vi "Indentation GUI - v4.vi"() -> ()   [LabVIEW 2013]
uses:
  Program Files (x86)/National Instruments/LabVIEW 2013/examples/Instrument IO/Serial/Serial - XON-XOFF Characters.ctl
  Program Files (x86)/National Instruments/LabVIEW 2013/examples/Instrument IO/Serial/Serial - ASCII Characters.ctl
  Program Files (x86)/National Instruments/LabVIEW 2013/examples/Instrument IO/Serial/Serial - Settings.ctl
  <vilib>/Instr/_visa.llb/VISA Configure Serial Port (Instr).vi
  <userlib>/DAQNavi Polymorphic VI/create/DAQNavi Create Channel(AI-Voltage).vi
  <userlib>/DAQNavi Polymorphic VI/read/DAQNavi Read (Analog DBL 1Chan 1Samp).vi
  <vilib>/Utility/file.llb/Write To Spreadsheet File (DBL).vi
panel:
  in  "offset":dbl
  in  "ground distance":dbl
  in  "contact":bool
  in  "停止 6":bool
  out "运动命令执行串口响应 4":string
  in  "终止符时结束读取？ 8":bool=TRUE
  in  "XON/XOFF字符 8":T1={"XON"=enum."DC1", "XOFF"=enum."DC3"}
  in  "终止符时结束写入？ 8":bool=TRUE
  in  "终止符 8":u8=10 format="%.0x"
  out "坐标设定命令串口传输响应 4":string
  in  "终止符时结束读取？ 7":bool=TRUE
  in  "XON/XOFF字符 7":T1={"XON"=enum."DC1", "XOFF"=enum."DC3"}
  in  "终止符时结束写入？ 7":bool=TRUE
  in  "终止符 7":u8=10 format="%.0x"
  in  "Fast Move":bool
  in  "停止 5":bool
  out "运动命令执行串口响应 3":string
  in  "终止符时结束读取？ 6":bool=TRUE
  in  "XON/XOFF字符 6":T1={"XON"=enum."DC1", "XOFF"=enum."DC3"}
  in  "终止符时结束写入？ 6":bool=TRUE
  in  "终止符 6":u8=10 format="%.0x"
  out "坐标设定命令串口传输响应 3":string
  in  "终止符时结束读取？ 5":bool=TRUE
  in  "XON/XOFF字符 5":T1={"XON"=enum."DC1", "XOFF"=enum."DC3"}
  in  "终止符时结束写入？ 5":bool=TRUE
  in  "终止符 5":u8=10 format="%.0x"
  in  "Backoff":bool
  in  "Sample+Slide":dbl
  in  "BaseLine":dbl=1.86
  in  "停止 4":bool
  out "运动命令执行串口响应 2":string
  in  "终止符时结束读取？ 4":bool=TRUE
  in  "XON/XOFF字符 4":T1={"XON"=enum."DC1", "XOFF"=enum."DC3"}
  in  "终止符时结束写入？ 4":bool=TRUE
  in  "终止符 4":u8=10 format="%.0x"
  out "Position setup command \nseries transport response 2":string
  in  "终止符时结束读取？ 3":bool=TRUE
  in  "XON/XOFF字符 3":T1={"XON"=enum."DC1", "XOFF"=enum."DC3"}
  in  "终止符时结束写入？ 3":bool=TRUE
  in  "终止符 3":u8=10 format="%.0x"
  out "Delay Counter":u64
  in  "indentation":bool
  in  "终止符 2":u8=10 format="%.0x"
  in  "终止符时结束写入？ 2":bool=TRUE
  in  "XON/XOFF字符 2":T1={"XON"=enum."DC1", "XOFF"=enum."DC3"}
  in  "终止符时结束读取？ 2":bool=TRUE
  out "Position setup command \nseries transport response":string
  in  "停止 3":bool
  out "Movement command execute \nseries transport response":string
  in  "停止 2":bool
  out "电压":cluster{"data":dbl, "data":dbl}(graph)
  out "data acquistion":bool
  in  "file path (dialog if empty)":path=path "C:/Users/user/Desktop/indentation data/新建 Microsoft Office Excel 工作表.xls" caption="文件路径 File Path"
  in  "Dwell Time (s)":dbl=180.0
  in  "Sample Frequency (Hz)":dbl=1000.0
  in  "Displacement (mm)":dbl
  in  "终止符时结束读取？":bool=TRUE
  in  "XON/XOFF字符":T1={"XON"=enum."DC1", "XOFF"=enum."DC3"}
  in  "终止符时结束写入？":bool=TRUE
  in  "终止符":u8=10 format="%.0x"
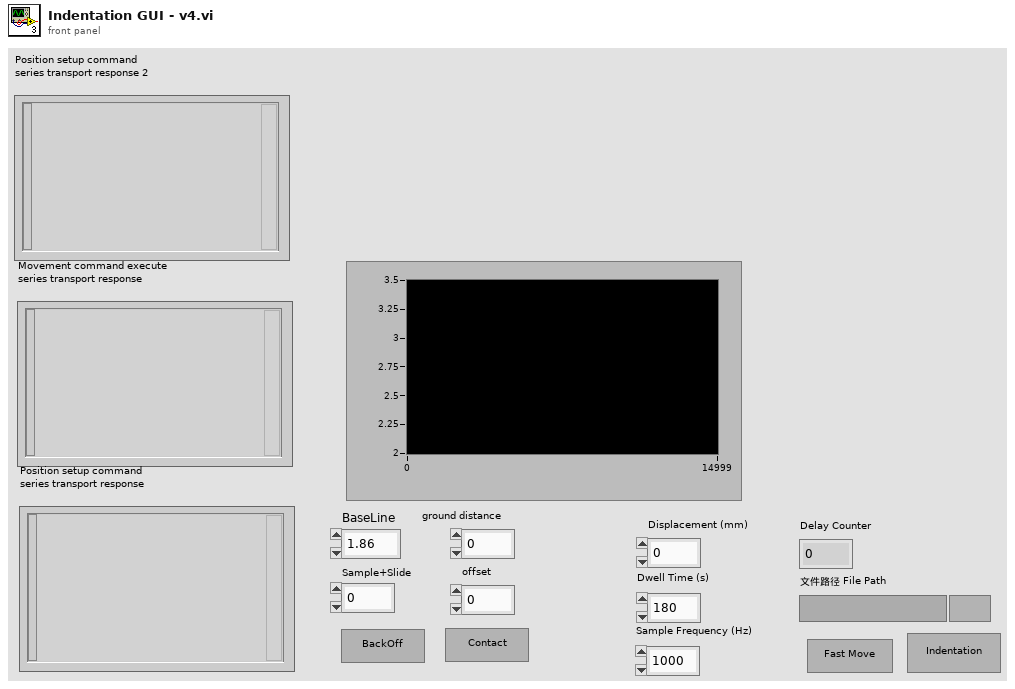
[diagram p1: front panel]
types:
  T1 = typedef "Serial - XON-XOFF Characters.ctl" = cluster{"XON":T2, "XOFF":T2}
  T2 = typedef "Serial - ASCII Characters.ctl" = enum16{"NUL", "SOH", "STX", "ETX", "EOT", "ENQ", "ACK", "BEL", "BS", "HT", "LF", "VT", "FF", "CR", "SO", "SI", "DLE", "DC1", "DC2", "DC3", "DC4", "NAK", "SYN", "ETB", "CAN", "EM", "SUB", "ESC", "FS", "GS", "RS", "US", "SP", "!", "\"", "#", "$", "%", "&", "'", "(", ")", "*", "+", ",", "- (-)", ".", "/", "0", "1", "2", "3", "4", "5", "6", "7", "8", "9", ":", ";", "<", "=", ">", "?", "@", "A", "B", "C", "D", "E", "F", "G", "H", "I", "J", "K", "L", "M", "N", "O", "P", "Q", "R", "S", "T", "U", "V", "W", "X", "Y", "Z", "[", "\\", "]", "^", "_", "`", "a", "b", "c", "d", "e", "f", "g", "h", "i", "j", "k", "l", "m", "n", "o", "p", "q", "r", "s", "t", "u", "v", "w", "x", "y", "z", "{", "|", "}", "~"}
  T3 = typedef "Serial - Settings.ctl" = cluster{"波特率":u32, "数据比特":u16, "奇偶":enum16{"None", "Odd", "Even", "Mark", "Space"}, "停止位":u16, "流控制":u16}
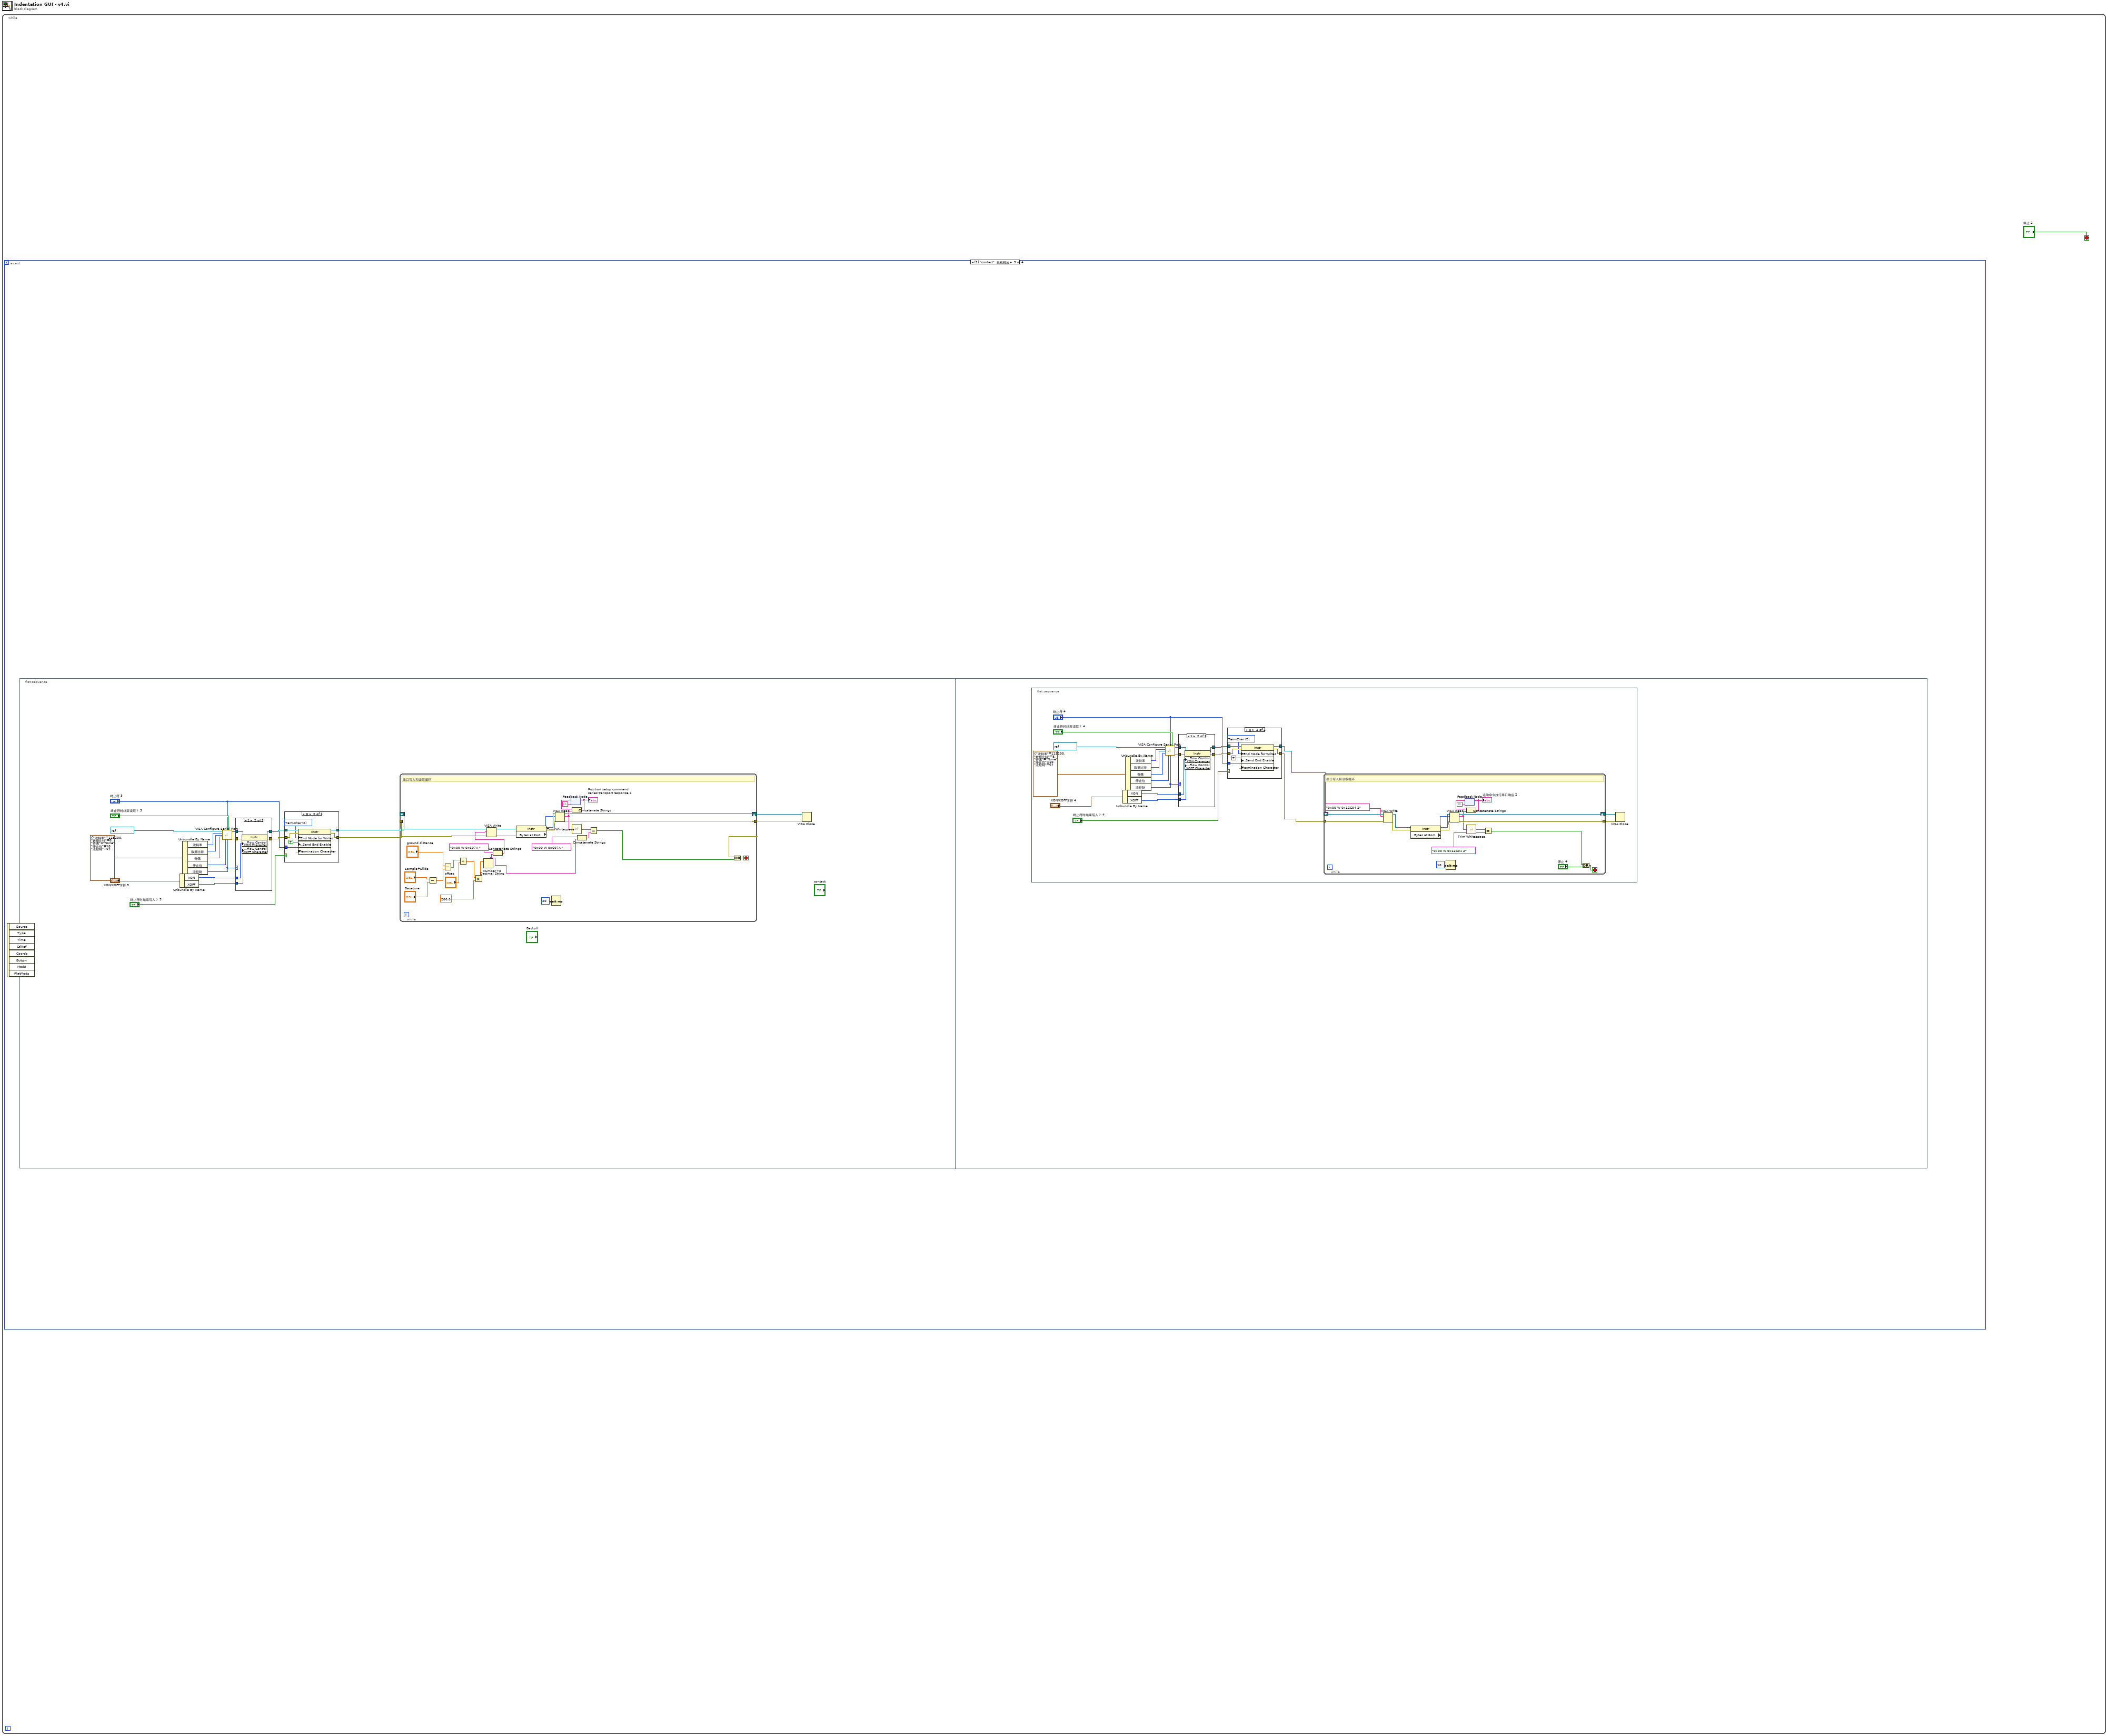
[diagram p0: block diagram]
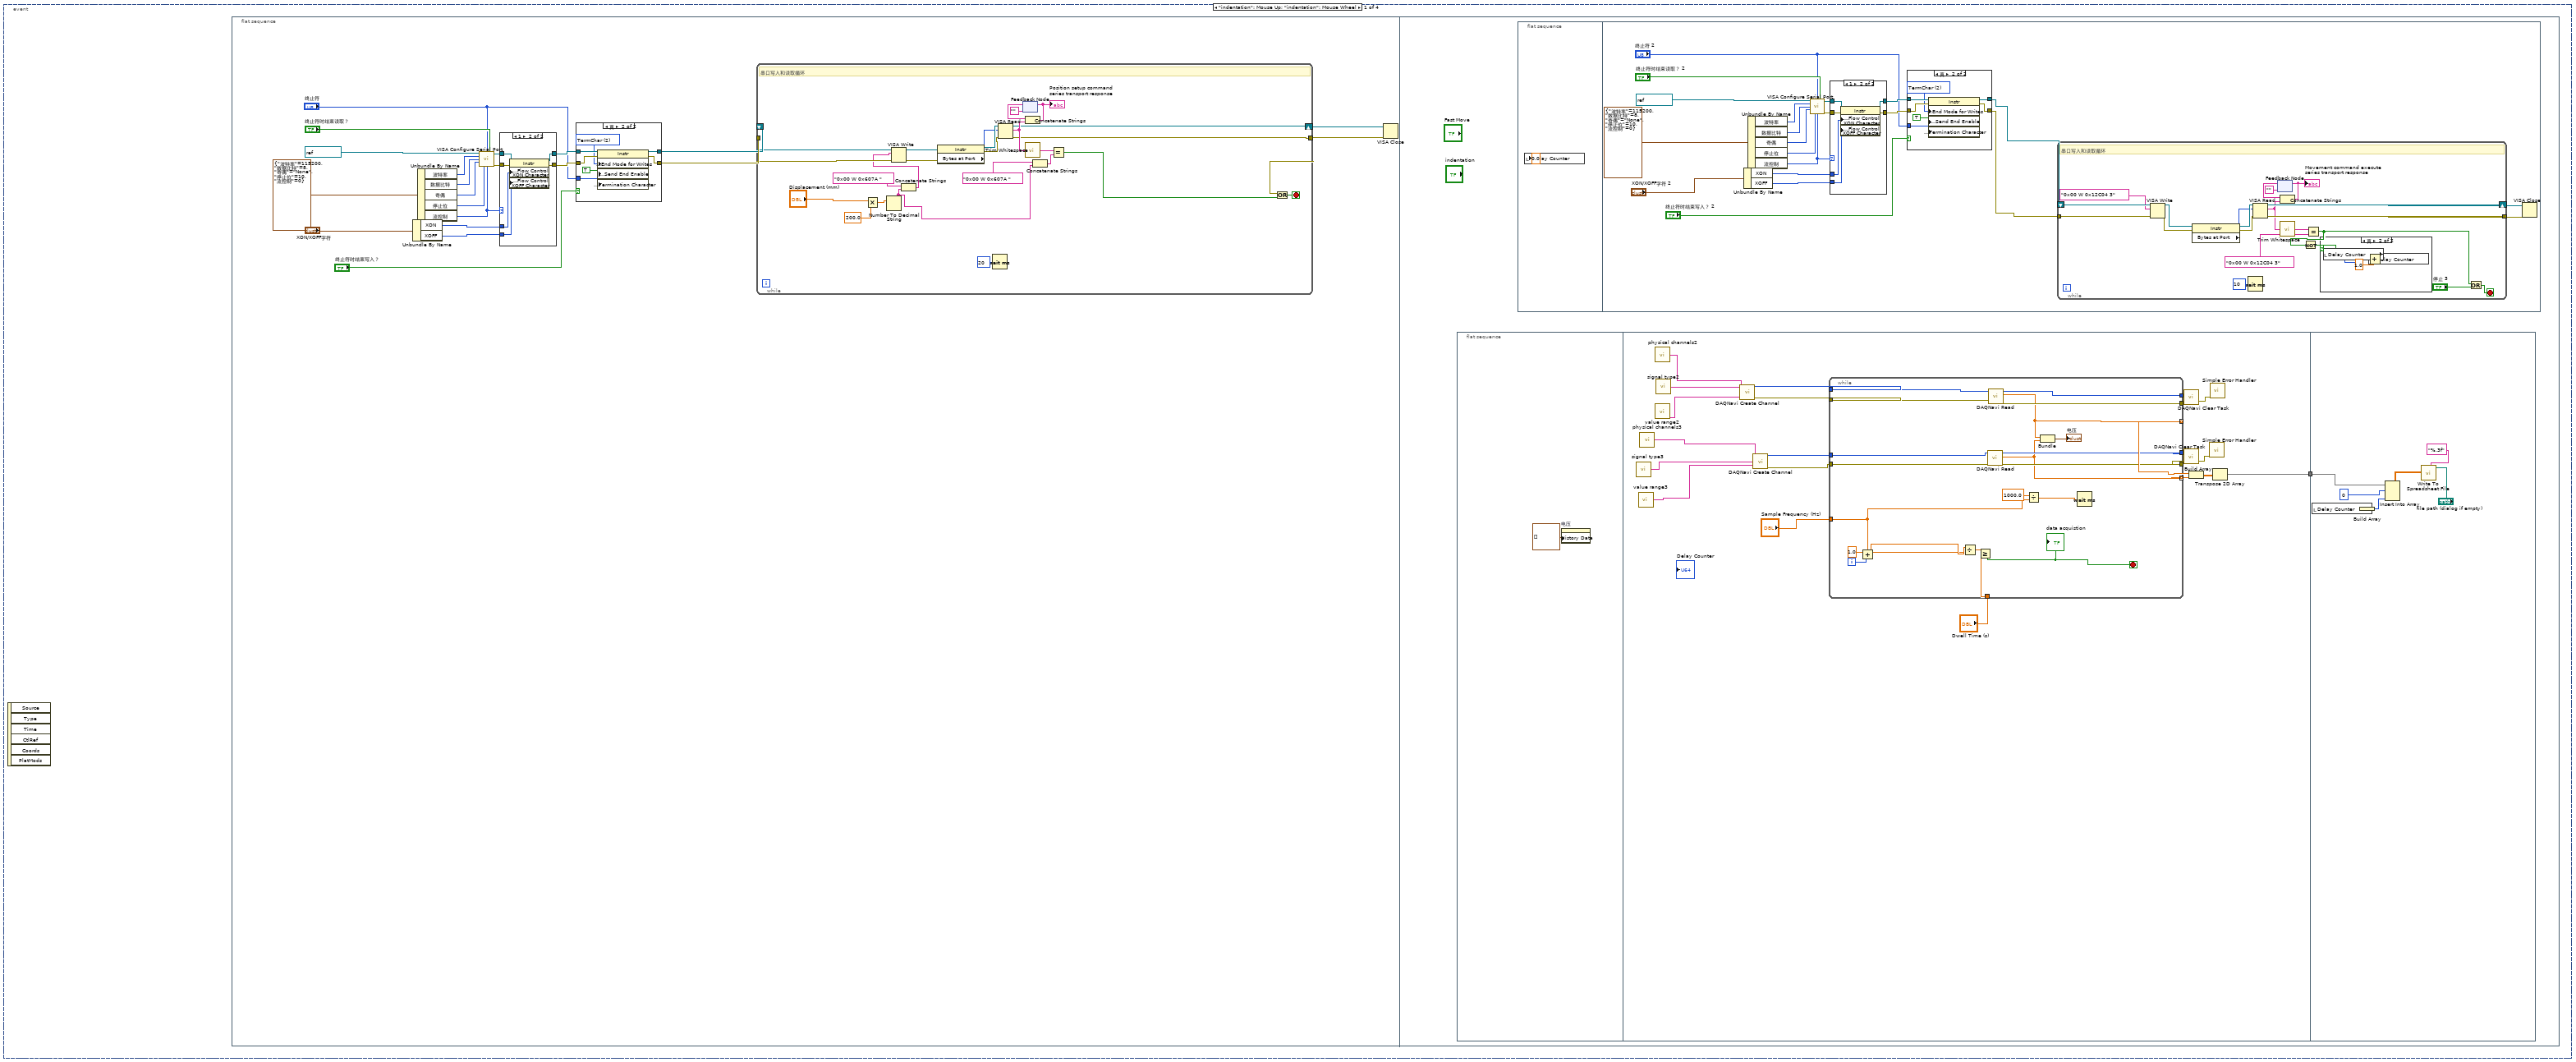
[diagram p2: hidden frame]
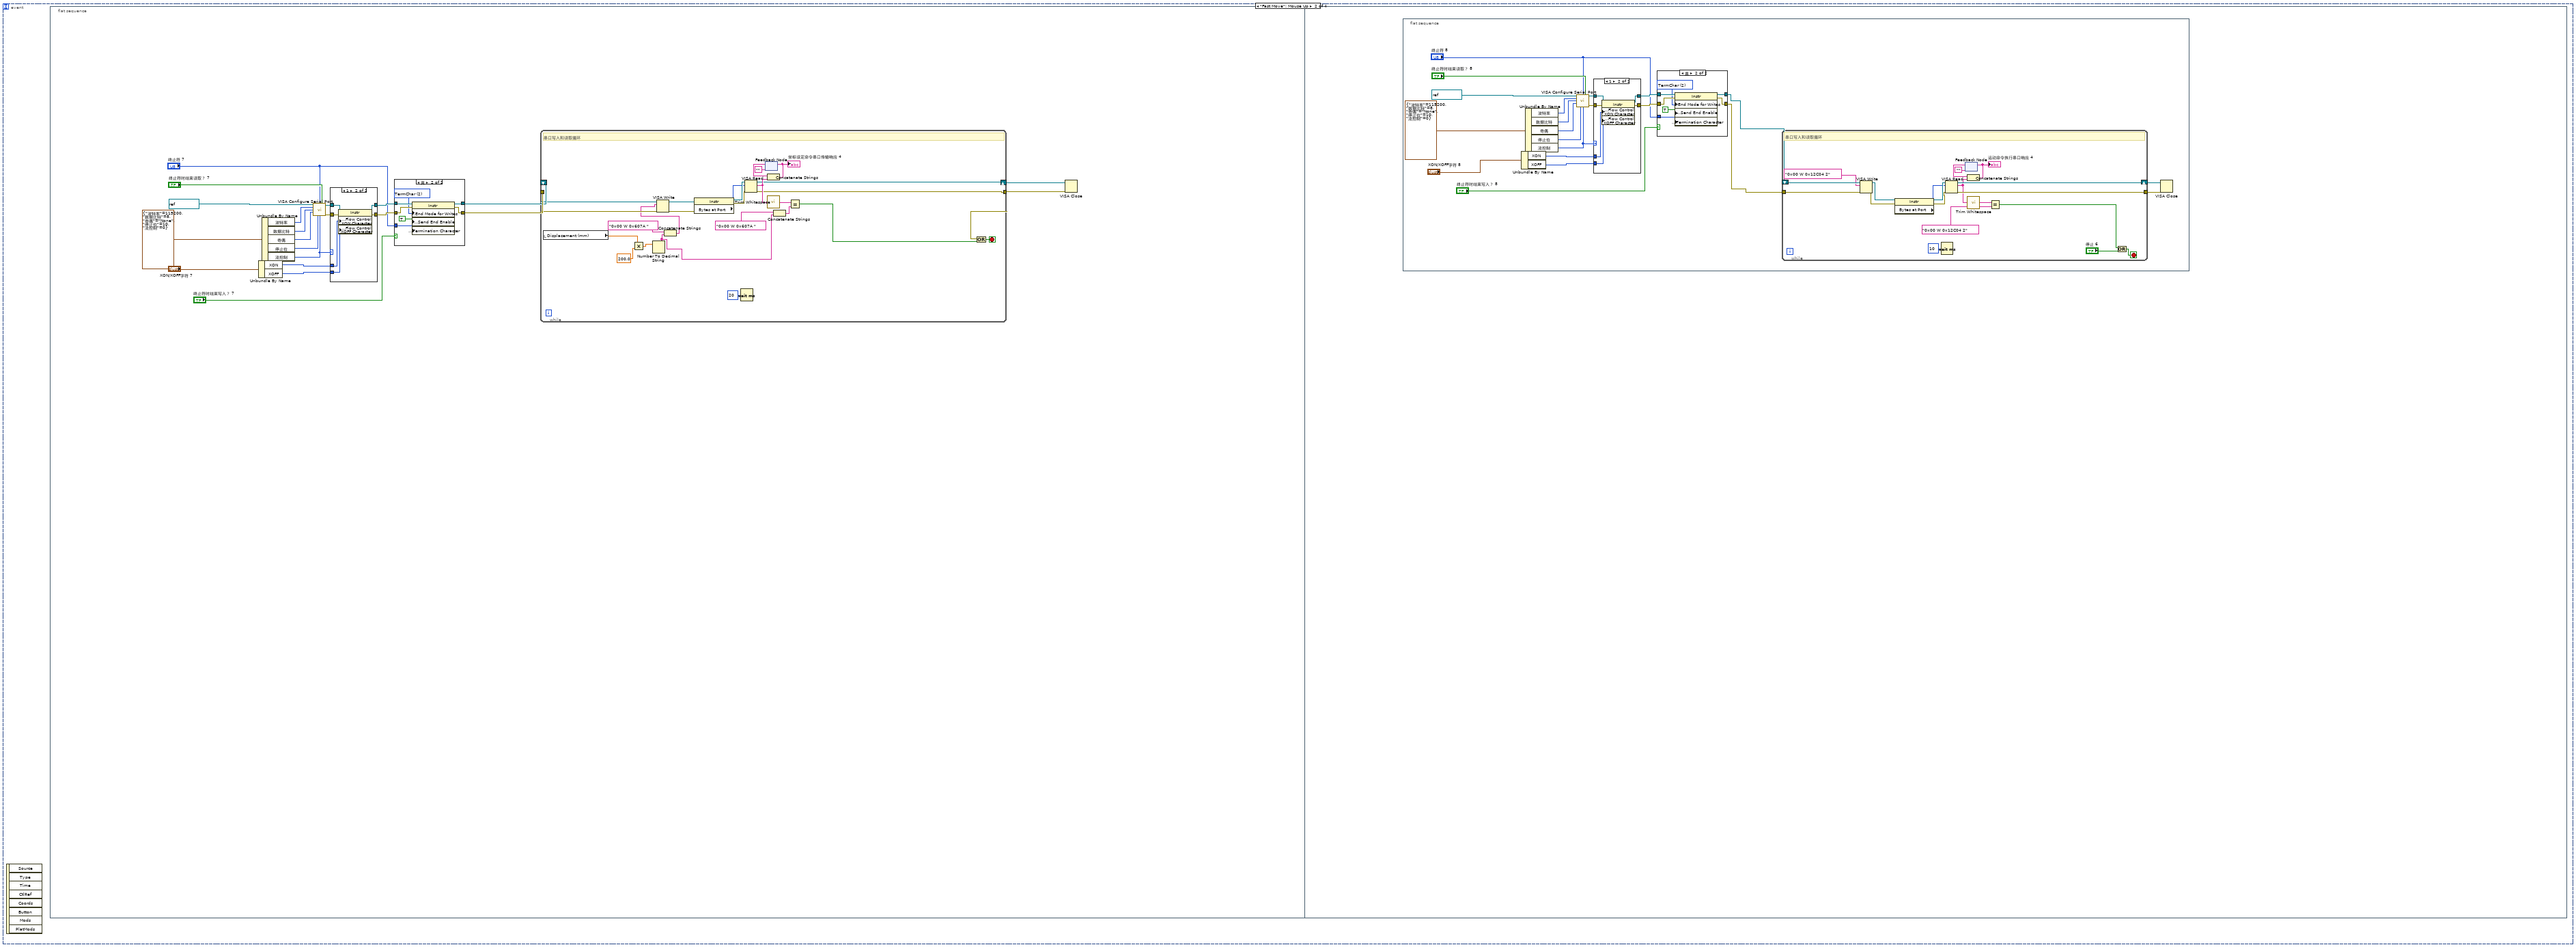
[diagram p8: hidden frame]
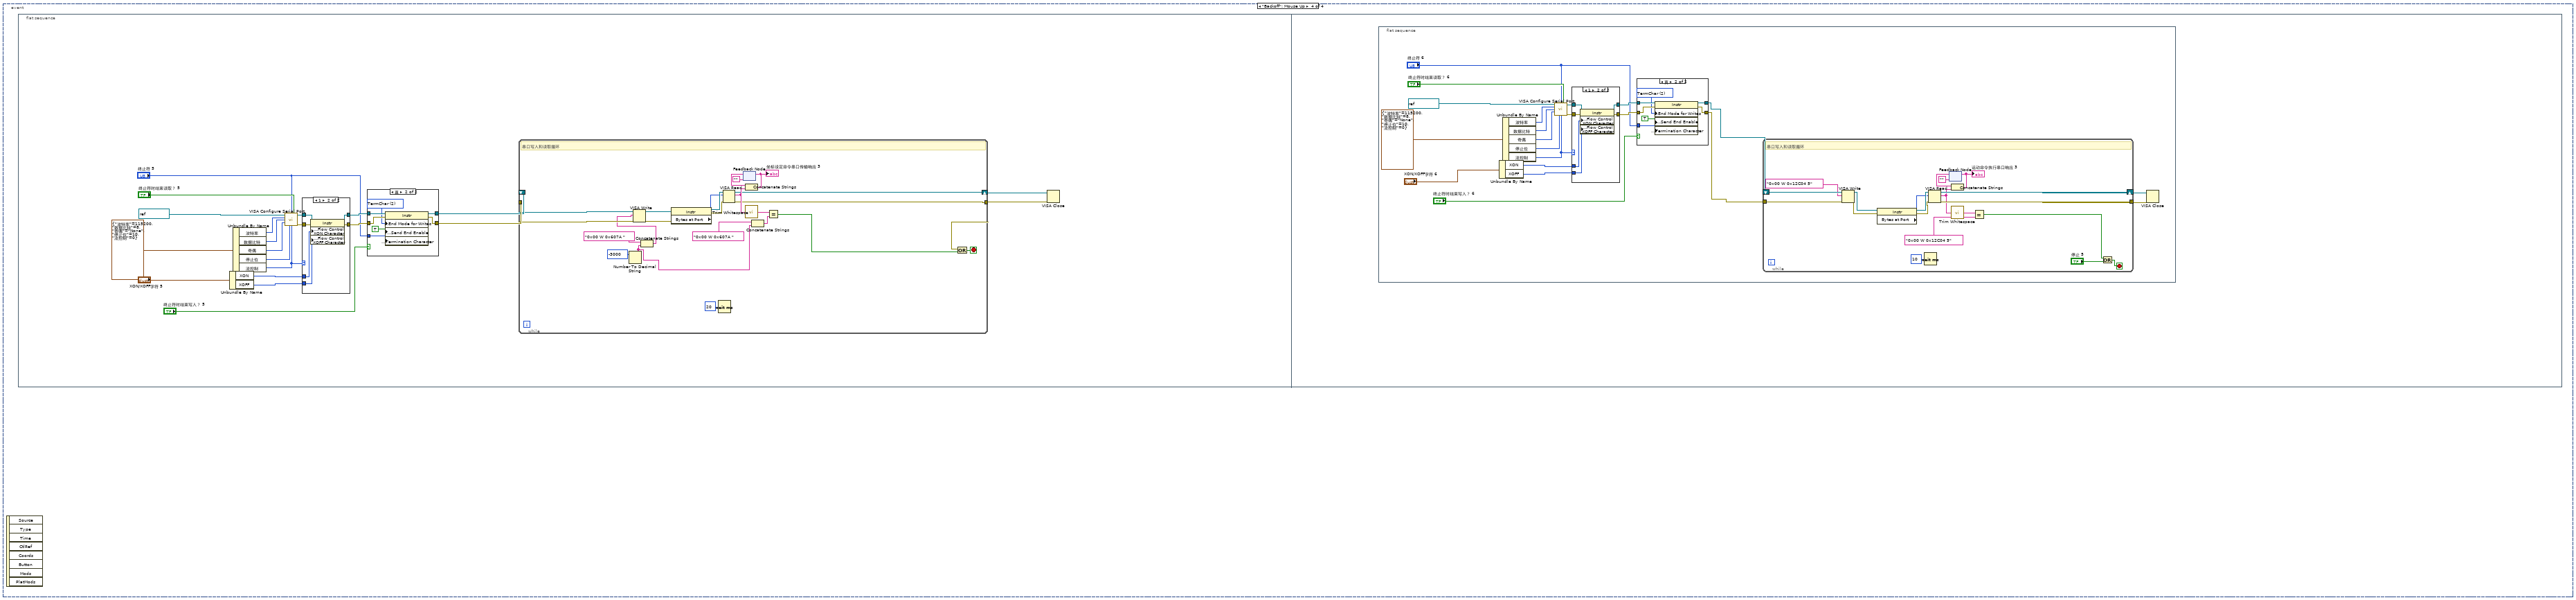
[diagram p17: hidden frame]
diagram:
  n1 = while {
    stop <- "停止 2" stop-if-true
    n2 = event shown="[2] \"contact\": 鼠标释放" {
      selector: _ -> [_ _ _ _]
      dyn-events: _ -> [_ _ _ _]
      timeout: _ -> [_ _ _ _]
      event "indentation": Mouse Up; "indentation": Mouse Wheel {
        n3 = event-data() -> ()  [unwired: 1 in, 6 out]
        n4 = flat-sequence {
          frame #0 {
            n5 = Unbundle By Name("XON/XOFF字符") -> ("XON"=w11:T2, "XOFF"=w10:T2)
            n6 = Unbundle By Name(T3 {"波特率"=115200, "数据比特"=8, "奇偶"=enum."None", "停止位"=10, "流控制"=0} ("串口设置")) -> ("波特率"=w15:u32, "数据比特"=w16:u16, "奇偶"=w17:enum16{"None", "Odd", "Even", "Mark", "Space"}, "停止位"=w18:u16, "流控制"=w12:u16)
            n7 = call-poly "VISA Configure Serial Port"("VISA resource name"=refnum<visa-resource-name> "COM3" ("VISA资源名称"), "termination char\n(0xA = '\\n' = LF)"="终止符", "Enable Termination\nChar (T)"="终止符时结束读取？", "baud rate (9600)"=w15, "data bits (8)"=w16, "parity (0:none)"=w17, "stop bits (10: 1 bit)"=w18, "flow control (0:none)"=w12) -> ("VISA resource name out"=w19:refnum<visa-resource-name>, "error out"=w20:errorcluster)  [unwired: 2 in, 4 out]
            n8 = case shown="1" w12 {
              tunnel: [w32 w39] -> w9
              tunnel: [w33 w38] -> w7
              tunnel: w20 -> [w32 w37]
              tunnel: w19 -> [w33 w36]
              tunnel: w11 -> [_ w35]
              tunnel: w10 -> [_ w34]
              frame Default {
              }
              frame 1 {
                n9 = property class="Instr"(reference=w36, error in=w37, "Serial Settings:Flow Control XON Character"=w35, "Serial Settings:Flow Control XOFF Character"=w34) -> (reference out=w38:refnum<visa-resource-name>, error out=w39:errorcluster)
              }
            }
            n10 = case shown="真" "终止符时结束写入？" {
              tunnel: w7 -> [w23 w31]
              tunnel: w9 -> [w24 w30]
              tunnel: [w23 w29] -> w6
              tunnel: [w24 w28] -> w8
              tunnel: "终止符" -> [_ w26]
              frame False {
              }
              frame True {
                w27 = u16 2 items=["None", "LastBit", "TermChar", "Break"] ("Serial Settings:Serial End Mode for Writes")
                n11 = property class="Instr"(reference=w31, error in=w30, "Serial Settings:End Mode for Writes"=w27, "Message Based Settings:Send End Enable"=TRUE, "Message Based Settings:Termination Character"=w26) -> (reference out=w29:refnum<visa-resource-name>, error out=w28:errorcluster)
              }
            }
            n12 = while {
              shift-right: [w47] -> w3
              shift-left: w6 -> [w63]
              tunnel: w8 -> [w62]
              tunnel: [w46] -> w2
              stop <- w64 stop-if-true
              # "串口写入和读取循环"
              n13 = Multiply(x="Displacement (mm)", y=200.0) -> (x*y=w59:dbl)
              n14 = Number To Decimal String(number=w59) -> (decimal integer string=w41:string)  [unwired: 1 in]
              n15 = Concatenate Strings("0x00 W 0x607A " ("字符串"), w41) -> (w57:string)
              n16 = VISA Write(VISA resource name=w63, write buffer=w57, error in (no error)=w62) -> (VISA resource name out=w44:refnum<visa-resource-name>, error out=w43:errorcluster)  [unwired: 1 out]
              n17 = property class="Instr"(reference=w44, error in=w43) -> (reference out=w52:refnum<visa-resource-name>, error out=w51:errorcluster, "Bytes at Port"=w50:u32)
              n18 = Wait (ms)(milliseconds to wait=u32 20 ("等待时间（毫秒）")) -> ()  [unwired: 1 out]
              n19 = VISA Read(VISA resource name=w52, byte count=w50, error in (no error)=w51) -> (VISA resource name out=w47:refnum<visa-resource-name>, read buffer=w49:string, error out=w46:errorcluster)  [unwired: 1 out]
              n20 = feedback #1("") -> (w55:string)
              n21 = Concatenate Strings(w55, w49) -> (w54:string)
              "Position setup command \nseries transport response" <- w54
              n22 = feedback-in #1(w54) -> ()
              n23 = call <vilib>:"Trim Whitespace.vi"("string"=w49) -> ("trimmed string"=w48:string)  [unwired: 1 in]
              n24 = Concatenate Strings("0x00 W 0x607A ", w41) -> (w40:string)
              n25 = Equal?(x=w48, y=w40) -> (x = y?=w45:bool)
              n26 = Or(x=w46, y=w45) -> (x .or. y?=w64:bool)
            }
            n27 = VISA Close(VISA resource name=w3, error in (no error)=w2) -> ()  [unwired: 1 out]
          }
          frame #1 {
            n28 = flat-sequence {
              tunnel: [w67] -> w65
              tunnel: w65 -> [w113]
              frame #0 {
                n29 = property on="电压" class="WFChart (严格)"("History Data"=cluster{"data":dbl, "data":dbl}[] [] ("历史数据")) -> ()  [unwired: 2 in, 2 out]
              }
              frame #1 {
                n30 = call "signal type3"() -> ("property value"=w79:string)  [unwired: 1 out]
                n31 = call "value range3"() -> ("property value"=w80:string)  [unwired: 1 out]
                n32 = call "physical channels3"() -> ("property value"=w78:string)  [unwired: 1 out]
                n33 = call "physical channels2"() -> ("property value"=w74:string)  [unwired: 1 out]
                n34 = call "value range2"() -> ("property value"=w75:string)  [unwired: 1 out]
                n35 = call "signal type2"() -> ("property value"=w68:string)  [unwired: 1 out]
                n36 = call-poly <userlib>:"DAQNavi Create Channel.vi"("physical channels"=w74, "signal type"=w68, "value range"=w75) -> ("task out"=w72:i32, "error out"=w71:errorcluster)  [unwired: 2 in, 9 out]
                n37 = call-poly <userlib>:"DAQNavi Create Channel.vi"("physical channels"=w78, "signal type"=w79, "value range"=w80) -> ("task out"=w76:i32, "error out"=w77:errorcluster)  [unwired: 11 in]
                n38 = while {
                  tunnel: w72 -> [w108]
                  tunnel: w71 -> [w107]
                  tunnel: [w106] -> w70
                  tunnel: [w105] -> w69
                  tunnel: w76 -> [w104]
                  tunnel: w77 -> [w103]
                  tunnel: [w102] -> w82
                  tunnel: [w101] -> w83
                  tunnel: [w97] -> w84 mode=indexing
                  tunnel: [w89] -> w85 mode=indexing
                  tunnel: "Dwell Time (s)" -> [w91]
                  tunnel: "Sample Frequency (Hz)" -> [w90]
                  i -> [w96]
                  stop <- w98 stop-if-true
                  n39 = Add(x=1.0, y=w96) -> (x+y=w94:dbl)
                  n40 = Divide(x=w94, y=w90) -> (x/y=w99:dbl)
                  n41 = Greater Or Equal?(x=w99, y=w91) -> (x >= y?=w98:bool)
                  "data acquistion" <- w98
                  n42 = call-poly <userlib>:"DAQNavi Read.vi"("error in (no error)"=w103, "task in"=w104) -> ("error out"=w101:errorcluster, "data"=w89:dbl, "task out"=w102:i32)  [unwired: 7 in]
                  n43 = call-poly <userlib>:"DAQNavi Read.vi"("error in (no error)"=w107, "task in"=w108) -> ("error out"=w105:errorcluster, "data"=w97:dbl, "task out"=w106:i32)  [unwired: 2 in, 5 out]
                  n44 = Divide(x=1000.0, y=w90) -> (x/y=w93:dbl)
                  n45 = Bundle("data"=w97, "data"=w89) -> (→"电压":cluster{"data":dbl, "data":dbl})  [unwired: 1 in]
                  n46 = Wait (ms)(milliseconds to wait=w93) -> ()  [unwired: 1 out]
                }
                n47 = call <userlib>:"DAQNavi Clear Task.vi"("error in (no error)"=w83, "task in"=w82) -> ("error out"=w81:errorcluster)  [unwired: 1 out]
                n48 = call <userlib>:"DAQNavi Clear Task.vi"("error in (no error)"=w69, "task in"=w70) -> ("error out"=w73:errorcluster)  [unwired: 1 out]
                n49 = Build Array(w84, w85) -> (w86:dbl[][])
                n50 = call <vilib>:"Simple Error Handler.vi"("error in (no error)"=w81) -> ()  [unwired: 2 in, 7 out]
                n51 = call <vilib>:"Simple Error Handler.vi"("error in (no error)"=w73) -> ()  [unwired: 2 in, 7 out]
                n52 = Transpose 2D Array(2D array=w86) -> (transposed array=w67:dbl[][])
              }
              frame #2 {
                n53 = local read "Delay Counter"() -> (w110:u64)
                n54 = Build Array(w110) -> (w109:u64[])
                n55 = Insert Into Array(array=w113, index (row)=0 ("索引 (行)"), new element=w109) -> (w111:dbl[][])  [unwired: 1 in]
                n56 = call-poly <vilib>:"Write To Spreadsheet File.vi"("format (%.3f)"="%.3f", "2D data"=w111, "file path (dialog if empty)"="file path (dialog if empty)") -> ()  [unwired: 5 in, 1 out]
              }
            }
            n57 = flat-sequence {
              frame #0 {
                n58 = local write "Delay Counter"(0.0 ("数值")) -> ()
              }
              frame #1 {
                n59 = Unbundle By Name("XON/XOFF字符 2") -> ("XON"=w124:T2, "XOFF"=w123:T2)
                n60 = Unbundle By Name(T3 {"波特率"=115200, "数据比特"=8, "奇偶"=enum."None", "停止位"=10, "流控制"=0} ("串口设置")) -> ("波特率"=w128:u32, "数据比特"=w129:u16, "奇偶"=w130:enum16{"None", "Odd", "Even", "Mark", "Space"}, "停止位"=w131:u16, "流控制"=w125:u16)
                n61 = call-poly "VISA Configure Serial Port"("VISA resource name"=refnum<visa-resource-name> "COM3" ("VISA资源名称"), "termination char\n(0xA = '\\n' = LF)"="终止符 2", "Enable Termination\nChar (T)"="终止符时结束读取？ 2", "baud rate (9600)"=w128, "data bits (8)"=w129, "parity (0:none)"=w130, "stop bits (10: 1 bit)"=w131, "flow control (0:none)"=w125) -> ("VISA resource name out"=w132:refnum<visa-resource-name>, "error out"=w133:errorcluster)  [unwired: 2 in, 4 out]
                n62 = case shown="1" w125 {
                  tunnel: [w147 w154] -> w122
                  tunnel: [w148 w153] -> w121
                  tunnel: w133 -> [w147 w152]
                  tunnel: w132 -> [w148 w151]
                  tunnel: w124 -> [_ w150]
                  tunnel: w123 -> [_ w149]
                  frame Default {
                  }
                  frame 1 {
                    n63 = property class="Instr"(reference=w151, error in=w152, "Serial Settings:Flow Control XON Character"=w150, "Serial Settings:Flow Control XOFF Character"=w149) -> (reference out=w153:refnum<visa-resource-name>, error out=w154:errorcluster)
                  }
                }
                n64 = case shown="真" "终止符时结束写入？ 2" {
                  tunnel: w121 -> [w138 w146]
                  tunnel: w122 -> [w139 w145]
                  tunnel: [w138 w144] -> w118
                  tunnel: [w139 w143] -> w117
                  tunnel: "终止符 2" -> [_ w141]
                  frame False {
                  }
                  frame True {
                    w142 = u16 2 items=["None", "LastBit", "TermChar", "Break"] ("Serial Settings:Serial End Mode for Writes")
                    n65 = property class="Instr"(reference=w146, error in=w145, "Serial Settings:End Mode for Writes"=w142, "Message Based Settings:Send End Enable"=TRUE, "Message Based Settings:Termination Character"=w141) -> (reference out=w144:refnum<visa-resource-name>, error out=w143:errorcluster)
                  }
                }
                n66 = while {
                  shift-right: [w175] -> w137
                  shift-left: w118 -> [w174]
                  tunnel: w117 -> [w173]
                  tunnel: [w171] -> w136
                  stop <- w160 stop-if-true
                  # "串口写入和读取循环"
                  n67 = VISA Write(VISA resource name=w174, write buffer="0x00 W 0x12C04 3" ("写入缓冲区"), error in (no error)=w173) -> (VISA resource name out=w165:refnum<visa-resource-name>, error out=w162:errorcluster)  [unwired: 1 out]
                  n68 = property class="Instr"(reference=w165, error in=w162) -> (reference out=w164:refnum<visa-resource-name>, error out=w163:errorcluster, "Bytes at Port"=w161:u32)
                  n69 = Wait (ms)(milliseconds to wait=u32 10) -> ()  [unwired: 1 out]
                  n70 = VISA Read(VISA resource name=w164, byte count=w161, error in (no error)=w163) -> (VISA resource name out=w175:refnum<visa-resource-name>, read buffer=w158:string, error out=w171:errorcluster)  [unwired: 1 out]
                  n71 = feedback #2("") -> (w169:string)
                  n72 = Concatenate Strings(w169, w158) -> (w168:string)
                  "Movement command execute \nseries transport response" <- w168
                  n73 = feedback-in #2(w168) -> ()
                  n74 = call <vilib>:"Trim Whitespace.vi"("string"=w158) -> ("trimmed string"=w157:string)  [unwired: 1 in]
                  n75 = Equal?(x=w157, y="0x00 W 0x12C04 3") -> (x = y?=w156:bool)
                  n76 = Not(x=w156) -> (.not. x?=w155:bool)
                  n77 = case shown="真" w155 {
                    frame False {
                    }
                    frame True {
                      n78 = local read "Delay Counter"() -> (w178:u64)
                      n79 = Add(x=w178, y=1.0) -> (x+y=w176:dbl)
                      n80 = local write "Delay Counter"(w176) -> ()
                    }
                  }
                  n81 = Or(x=w156, y="停止 3") -> (x .or. y?=w160:bool)
                }
                n82 = VISA Close(VISA resource name=w137, error in (no error)=w136) -> ()  [unwired: 1 out]
              }
            }
          }
        }
      }
      event "Fast Move": Mouse Up {
        n83 = event-data() -> ()  [unwired: 1 in, 8 out]
        n84 = flat-sequence {
          frame #0 {
            n85 = Unbundle By Name("XON/XOFF字符 7") -> ("XON"=w188:T2, "XOFF"=w187:T2)
            n86 = Unbundle By Name(T3 {"波特率"=115200, "数据比特"=8, "奇偶"=enum."None", "停止位"=10, "流控制"=0} ("串口设置")) -> ("波特率"=w192:u32, "数据比特"=w193:u16, "奇偶"=w194:enum16{"None", "Odd", "Even", "Mark", "Space"}, "停止位"=w195:u16, "流控制"=w189:u16)
            n87 = call-poly "VISA Configure Serial Port"("VISA resource name"=refnum<visa-resource-name> "COM3" ("VISA资源名称"), "termination char\n(0xA = '\\n' = LF)"="终止符 7", "Enable Termination\nChar (T)"="终止符时结束读取？ 7", "baud rate (9600)"=w192, "data bits (8)"=w193, "parity (0:none)"=w194, "stop bits (10: 1 bit)"=w195, "flow control (0:none)"=w189) -> ("VISA resource name out"=w196:refnum<visa-resource-name>, "error out"=w197:errorcluster)  [unwired: 2 in, 4 out]
            n88 = case shown="1" w189 {
              tunnel: [w209 w216] -> w186
              tunnel: [w210 w215] -> w184
              tunnel: w197 -> [w209 w214]
              tunnel: w196 -> [w210 w213]
              tunnel: w188 -> [_ w212]
              tunnel: w187 -> [_ w211]
              frame Default {
              }
              frame 1 {
                n89 = property class="Instr"(reference=w213, error in=w214, "Serial Settings:Flow Control XON Character"=w212, "Serial Settings:Flow Control XOFF Character"=w211) -> (reference out=w215:refnum<visa-resource-name>, error out=w216:errorcluster)
              }
            }
            n90 = case shown="真" "终止符时结束写入？ 7" {
              tunnel: w184 -> [w200 w208]
              tunnel: w186 -> [w201 w207]
              tunnel: [w200 w206] -> w183
              tunnel: [w201 w205] -> w185
              tunnel: "终止符 7" -> [_ w203]
              frame False {
              }
              frame True {
                w204 = u16 2 items=["None", "LastBit", "TermChar", "Break"] ("Serial Settings:Serial End Mode for Writes")
                n91 = property class="Instr"(reference=w208, error in=w207, "Serial Settings:End Mode for Writes"=w204, "Message Based Settings:Send End Enable"=TRUE, "Message Based Settings:Termination Character"=w203) -> (reference out=w206:refnum<visa-resource-name>, error out=w205:errorcluster)
              }
            }
            n92 = while {
              shift-right: [w227] -> w180
              shift-left: w183 -> [w240]
              tunnel: w185 -> [w239]
              tunnel: [w226] -> w179
              stop <- w241 stop-if-true
              # "串口写入和读取循环"
              n93 = local read "Displacement (mm)"() -> (w219:dbl)
              n94 = Multiply(x=w219, y=200.0) -> (x*y=w217:dbl)
              n95 = Number To Decimal String(number=w217) -> (decimal integer string=w221:string)  [unwired: 1 in]
              n96 = Concatenate Strings("0x00 W 0x607A " ("字符串"), w221) -> (w237:string)
              n97 = VISA Write(VISA resource name=w240, write buffer=w237, error in (no error)=w239) -> (VISA resource name out=w224:refnum<visa-resource-name>, error out=w223:errorcluster)  [unwired: 1 out]
              n98 = property class="Instr"(reference=w224, error in=w223) -> (reference out=w232:refnum<visa-resource-name>, error out=w231:errorcluster, "Bytes at Port"=w230:u32)
              n99 = Wait (ms)(milliseconds to wait=u32 20 ("等待时间（毫秒）")) -> ()  [unwired: 1 out]
              n100 = VISA Read(VISA resource name=w232, byte count=w230, error in (no error)=w231) -> (VISA resource name out=w227:refnum<visa-resource-name>, read buffer=w229:string, error out=w226:errorcluster)  [unwired: 1 out]
              n101 = feedback #3("") -> (w235:string)
              n102 = Concatenate Strings(w235, w229) -> (w234:string)
              "坐标设定命令串口传输响应 4" <- w234
              n103 = feedback-in #3(w234) -> ()
              n104 = call <vilib>:"Trim Whitespace.vi"("string"=w229) -> ("trimmed string"=w228:string)  [unwired: 1 in]
              n105 = Concatenate Strings("0x00 W 0x607A ", w221) -> (w220:string)
              n106 = Equal?(x=w228, y=w220) -> (x = y?=w225:bool)
              n107 = Or(x=w226, y=w225) -> (x .or. y?=w241:bool)
            }
            n108 = VISA Close(VISA resource name=w180, error in (no error)=w179) -> ()  [unwired: 1 out]
          }
          frame #1 {
            n109 = flat-sequence {
              frame #0 {
                n110 = Unbundle By Name("XON/XOFF字符 8") -> ("XON"=w249:T2, "XOFF"=w248:T2)
                n111 = Unbundle By Name(T3 {"波特率"=115200, "数据比特"=8, "奇偶"=enum."None", "停止位"=10, "流控制"=0} ("串口设置")) -> ("波特率"=w253:u32, "数据比特"=w254:u16, "奇偶"=w255:enum16{"None", "Odd", "Even", "Mark", "Space"}, "停止位"=w256:u16, "流控制"=w250:u16)
                n112 = call-poly "VISA Configure Serial Port"("VISA resource name"=refnum<visa-resource-name> "COM3" ("VISA资源名称"), "termination char\n(0xA = '\\n' = LF)"="终止符 8", "Enable Termination\nChar (T)"="终止符时结束读取？ 8", "baud rate (9600)"=w253, "data bits (8)"=w254, "parity (0:none)"=w255, "stop bits (10: 1 bit)"=w256, "flow control (0:none)"=w250) -> ("VISA resource name out"=w257:refnum<visa-resource-name>, "error out"=w258:errorcluster)  [unwired: 2 in, 4 out]
                n113 = case shown="1" w250 {
                  tunnel: [w272 w279] -> w247
                  tunnel: [w273 w278] -> w246
                  tunnel: w258 -> [w272 w277]
                  tunnel: w257 -> [w273 w276]
                  tunnel: w249 -> [_ w275]
                  tunnel: w248 -> [_ w274]
                  frame Default {
                  }
                  frame 1 {
                    n114 = property class="Instr"(reference=w276, error in=w277, "Serial Settings:Flow Control XON Character"=w275, "Serial Settings:Flow Control XOFF Character"=w274) -> (reference out=w278:refnum<visa-resource-name>, error out=w279:errorcluster)
                  }
                }
                n115 = case shown="真" "终止符时结束写入？ 8" {
                  tunnel: w246 -> [w263 w271]
                  tunnel: w247 -> [w264 w270]
                  tunnel: [w263 w269] -> w243
                  tunnel: [w264 w268] -> w242
                  tunnel: "终止符 8" -> [_ w266]
                  frame False {
                  }
                  frame True {
                    w267 = u16 2 items=["None", "LastBit", "TermChar", "Break"] ("Serial Settings:Serial End Mode for Writes")
                    n116 = property class="Instr"(reference=w271, error in=w270, "Serial Settings:End Mode for Writes"=w267, "Message Based Settings:Send End Enable"=TRUE, "Message Based Settings:Termination Character"=w266) -> (reference out=w269:refnum<visa-resource-name>, error out=w268:errorcluster)
                  }
                }
                n117 = while {
                  shift-right: [w299] -> w262
                  shift-left: w243 -> [w298]
                  tunnel: w242 -> [w297]
                  tunnel: [w295] -> w261
                  stop <- w284 stop-if-true
                  # "串口写入和读取循环"
                  n118 = VISA Write(VISA resource name=w298, write buffer="0x00 W 0x12C04 2" ("写入缓冲区"), error in (no error)=w297) -> (VISA resource name out=w289:refnum<visa-resource-name>, error out=w286:errorcluster)  [unwired: 1 out]
                  n119 = property class="Instr"(reference=w289, error in=w286) -> (reference out=w288:refnum<visa-resource-name>, error out=w287:errorcluster, "Bytes at Port"=w285:u32)
                  n120 = Wait (ms)(milliseconds to wait=u32 10) -> ()  [unwired: 1 out]
                  n121 = VISA Read(VISA resource name=w288, byte count=w285, error in (no error)=w287) -> (VISA resource name out=w299:refnum<visa-resource-name>, read buffer=w282:string, error out=w295:errorcluster)  [unwired: 1 out]
                  n122 = feedback #4("") -> (w293:string)
                  n123 = Concatenate Strings(w293, w282) -> (w292:string)
                  "运动命令执行串口响应 4" <- w292
                  n124 = feedback-in #4(w292) -> ()
                  n125 = call <vilib>:"Trim Whitespace.vi"("string"=w282) -> ("trimmed string"=w281:string)  [unwired: 1 in]
                  n126 = Equal?(x=w281, y="0x00 W 0x12C04 2") -> (x = y?=w280:bool)
                  n127 = Or(x=w280, y="停止 6") -> (x .or. y?=w284:bool)
                }
                n128 = VISA Close(VISA resource name=w262, error in (no error)=w261) -> ()  [unwired: 1 out]
              }
            }
          }
        }
      }
      event "contact": Mouse Up {
        n129 = event-data() -> ()  [unwired: 1 in, 8 out]
        n130 = flat-sequence {
          frame #0 {
            n131 = Unbundle By Name("XON/XOFF字符 3") -> ("XON"=w309:T2, "XOFF"=w308:T2)
            n132 = Unbundle By Name(T3 {"波特率"=115200, "数据比特"=8, "奇偶"=enum."None", "停止位"=10, "流控制"=0} ("串口设置")) -> ("波特率"=w313:u32, "数据比特"=w314:u16, "奇偶"=w315:enum16{"None", "Odd", "Even", "Mark", "Space"}, "停止位"=w316:u16, "流控制"=w310:u16)
            n133 = call-poly "VISA Configure Serial Port"("VISA resource name"=refnum<visa-resource-name> "COM3" ("VISA资源名称"), "termination char\n(0xA = '\\n' = LF)"="终止符 3", "Enable Termination\nChar (T)"="终止符时结束读取？ 3", "baud rate (9600)"=w313, "data bits (8)"=w314, "parity (0:none)"=w315, "stop bits (10: 1 bit)"=w316, "flow control (0:none)"=w310) -> ("VISA resource name out"=w317:refnum<visa-resource-name>, "error out"=w318:errorcluster)  [unwired: 2 in, 4 out]
            n134 = case shown="1" w310 {
              tunnel: [w330 w337] -> w307
              tunnel: [w331 w336] -> w305
              tunnel: w318 -> [w330 w335]
              tunnel: w317 -> [w331 w334]
              tunnel: w309 -> [_ w333]
              tunnel: w308 -> [_ w332]
              frame Default {
              }
              frame 1 {
                n135 = property class="Instr"(reference=w334, error in=w335, "Serial Settings:Flow Control XON Character"=w333, "Serial Settings:Flow Control XOFF Character"=w332) -> (reference out=w336:refnum<visa-resource-name>, error out=w337:errorcluster)
              }
            }
            n136 = case shown="真" "终止符时结束写入？ 3" {
              tunnel: w305 -> [w321 w329]
              tunnel: w307 -> [w322 w328]
              tunnel: [w321 w327] -> w304
              tunnel: [w322 w326] -> w306
              tunnel: "终止符 3" -> [_ w324]
              frame False {
              }
              frame True {
                w325 = u16 2 items=["None", "LastBit", "TermChar", "Break"] ("Serial Settings:Serial End Mode for Writes")
                n137 = property class="Instr"(reference=w329, error in=w328, "Serial Settings:End Mode for Writes"=w325, "Message Based Settings:Send End Enable"=TRUE, "Message Based Settings:Termination Character"=w324) -> (reference out=w327:refnum<visa-resource-name>, error out=w326:errorcluster)
              }
            }
            n138 = while {
              shift-right: [w353] -> w301
              shift-left: w304 -> [w367]
              tunnel: w306 -> [w366]
              tunnel: [w352] -> w300
              stop <- w368 stop-if-true
              # "串口写入和读取循环"
              n139 = Subtract(x="Sample+Slide", y="BaseLine") -> (x-y=w343:dbl)
              n140 = Subtract(x="ground distance", y=w343) -> (x-y=w340:dbl)
              n141 = Add(x=w340, y="offset") -> (x+y=w338:dbl)
              n142 = Multiply(x=w338, y=200.0) -> (x*y=w342:dbl)
              n143 = Number To Decimal String(number=w342) -> (decimal integer string=w347:string)  [unwired: 1 in]
              n144 = Concatenate Strings("0x00 W 0x607A " ("字符串"), w347) -> (w363:string)
              n145 = VISA Write(VISA resource name=w367, write buffer=w363, error in (no error)=w366) -> (VISA resource name out=w350:refnum<visa-resource-name>, error out=w349:errorcluster)  [unwired: 1 out]
              n146 = property class="Instr"(reference=w350, error in=w349) -> (reference out=w358:refnum<visa-resource-name>, error out=w357:errorcluster, "Bytes at Port"=w356:u32)
              n147 = Wait (ms)(milliseconds to wait=u32 20 ("等待时间（毫秒）")) -> ()  [unwired: 1 out]
              n148 = VISA Read(VISA resource name=w358, byte count=w356, error in (no error)=w357) -> (VISA resource name out=w353:refnum<visa-resource-name>, read buffer=w355:string, error out=w352:errorcluster)  [unwired: 1 out]
              n149 = feedback #5("") -> (w361:string)
              n150 = Concatenate Strings(w361, w355) -> (w360:string)
              "Position setup command \nseries transport response 2" <- w360
              n151 = feedback-in #5(w360) -> ()
              n152 = call <vilib>:"Trim Whitespace.vi"("string"=w355) -> ("trimmed string"=w354:string)  [unwired: 1 in]
              n153 = Concatenate Strings("0x00 W 0x607A ", w347) -> (w346:string)
              n154 = Equal?(x=w354, y=w346) -> (x = y?=w351:bool)
              n155 = Or(x=w352, y=w351) -> (x .or. y?=w368:bool)
            }
            n156 = VISA Close(VISA resource name=w301, error in (no error)=w300) -> ()  [unwired: 1 out]
          }
          frame #1 {
            n157 = flat-sequence {
              frame #0 {
                n158 = Unbundle By Name("XON/XOFF字符 4") -> ("XON"=w376:T2, "XOFF"=w375:T2)
                n159 = Unbundle By Name(T3 {"波特率"=115200, "数据比特"=8, "奇偶"=enum."None", "停止位"=10, "流控制"=0} ("串口设置")) -> ("波特率"=w380:u32, "数据比特"=w381:u16, "奇偶"=w382:enum16{"None", "Odd", "Even", "Mark", "Space"}, "停止位"=w383:u16, "流控制"=w377:u16)
                n160 = call-poly "VISA Configure Serial Port"("VISA resource name"=refnum<visa-resource-name> "COM3" ("VISA资源名称"), "termination char\n(0xA = '\\n' = LF)"="终止符 4", "Enable Termination\nChar (T)"="终止符时结束读取？ 4", "baud rate (9600)"=w380, "data bits (8)"=w381, "parity (0:none)"=w382, "stop bits (10: 1 bit)"=w383, "flow control (0:none)"=w377) -> ("VISA resource name out"=w384:refnum<visa-resource-name>, "error out"=w385:errorcluster)  [unwired: 2 in, 4 out]
                n161 = case shown="1" w377 {
                  tunnel: [w399 w406] -> w374
                  tunnel: [w400 w405] -> w373
                  tunnel: w385 -> [w399 w404]
                  tunnel: w384 -> [w400 w403]
                  tunnel: w376 -> [_ w402]
                  tunnel: w375 -> [_ w401]
                  frame Default {
                  }
                  frame 1 {
                    n162 = property class="Instr"(reference=w403, error in=w404, "Serial Settings:Flow Control XON Character"=w402, "Serial Settings:Flow Control XOFF Character"=w401) -> (reference out=w405:refnum<visa-resource-name>, error out=w406:errorcluster)
                  }
                }
                n163 = case shown="真" "终止符时结束写入？ 4" {
                  tunnel: w373 -> [w390 w398]
                  tunnel: w374 -> [w391 w397]
                  tunnel: [w390 w396] -> w370
                  tunnel: [w391 w395] -> w369
                  tunnel: "终止符 4" -> [_ w393]
                  frame False {
                  }
                  frame True {
                    w394 = u16 2 items=["None", "LastBit", "TermChar", "Break"] ("Serial Settings:Serial End Mode for Writes")
                    n164 = property class="Instr"(reference=w398, error in=w397, "Serial Settings:End Mode for Writes"=w394, "Message Based Settings:Send End Enable"=TRUE, "Message Based Settings:Termination Character"=w393) -> (reference out=w396:refnum<visa-resource-name>, error out=w395:errorcluster)
                  }
                }
                n165 = while {
                  shift-right: [w426] -> w389
                  shift-left: w370 -> [w425]
                  tunnel: w369 -> [w424]
                  tunnel: [w422] -> w388
                  stop <- w411 stop-if-true
                  # "串口写入和读取循环"
                  n166 = VISA Write(VISA resource name=w425, write buffer="0x00 W 0x12C04 2" ("写入缓冲区"), error in (no error)=w424) -> (VISA resource name out=w416:refnum<visa-resource-name>, error out=w413:errorcluster)  [unwired: 1 out]
                  n167 = property class="Instr"(reference=w416, error in=w413) -> (reference out=w415:refnum<visa-resource-name>, error out=w414:errorcluster, "Bytes at Port"=w412:u32)
                  n168 = Wait (ms)(milliseconds to wait=u32 10) -> ()  [unwired: 1 out]
                  n169 = VISA Read(VISA resource name=w415, byte count=w412, error in (no error)=w414) -> (VISA resource name out=w426:refnum<visa-resource-name>, read buffer=w409:string, error out=w422:errorcluster)  [unwired: 1 out]
                  n170 = feedback #6("") -> (w420:string)
                  n171 = Concatenate Strings(w420, w409) -> (w419:string)
                  "运动命令执行串口响应 2" <- w419
                  n172 = feedback-in #6(w419) -> ()
                  n173 = call <vilib>:"Trim Whitespace.vi"("string"=w409) -> ("trimmed string"=w408:string)  [unwired: 1 in]
                  n174 = Equal?(x=w408, y="0x00 W 0x12C04 2") -> (x = y?=w407:bool)
                  n175 = Or(x=w407, y="停止 4") -> (x .or. y?=w411:bool)
                }
                n176 = VISA Close(VISA resource name=w389, error in (no error)=w388) -> ()  [unwired: 1 out]
              }
            }
          }
        }
      }
      event "Backoff": Mouse Up {
        n177 = event-data() -> ()  [unwired: 1 in, 8 out]
        n178 = flat-sequence {
          frame #0 {
            n179 = Unbundle By Name("XON/XOFF字符 5") -> ("XON"=w436:T2, "XOFF"=w435:T2)
            n180 = Unbundle By Name(T3 {"波特率"=115200, "数据比特"=8, "奇偶"=enum."None", "停止位"=10, "流控制"=0} ("串口设置")) -> ("波特率"=w440:u32, "数据比特"=w441:u16, "奇偶"=w442:enum16{"None", "Odd", "Even", "Mark", "Space"}, "停止位"=w443:u16, "流控制"=w437:u16)
            n181 = call-poly "VISA Configure Serial Port"("VISA resource name"=refnum<visa-resource-name> "COM3" ("VISA资源名称"), "termination char\n(0xA = '\\n' = LF)"="终止符 5", "Enable Termination\nChar (T)"="终止符时结束读取？ 5", "baud rate (9600)"=w440, "data bits (8)"=w441, "parity (0:none)"=w442, "stop bits (10: 1 bit)"=w443, "flow control (0:none)"=w437) -> ("VISA resource name out"=w444:refnum<visa-resource-name>, "error out"=w445:errorcluster)  [unwired: 2 in, 4 out]
            n182 = case shown="1" w437 {
              tunnel: [w457 w464] -> w434
              tunnel: [w458 w463] -> w432
              tunnel: w445 -> [w457 w462]
              tunnel: w444 -> [w458 w461]
              tunnel: w436 -> [_ w460]
              tunnel: w435 -> [_ w459]
              frame Default {
              }
              frame 1 {
                n183 = property class="Instr"(reference=w461, error in=w462, "Serial Settings:Flow Control XON Character"=w460, "Serial Settings:Flow Control XOFF Character"=w459) -> (reference out=w463:refnum<visa-resource-name>, error out=w464:errorcluster)
              }
            }
            n184 = case shown="真" "终止符时结束写入？ 5" {
              tunnel: w432 -> [w448 w456]
              tunnel: w434 -> [w449 w455]
              tunnel: [w448 w454] -> w431
              tunnel: [w449 w453] -> w433
              tunnel: "终止符 5" -> [_ w451]
              frame False {
              }
              frame True {
                w452 = u16 2 items=["None", "LastBit", "TermChar", "Break"] ("Serial Settings:Serial End Mode for Writes")
                n185 = property class="Instr"(reference=w456, error in=w455, "Serial Settings:End Mode for Writes"=w452, "Message Based Settings:Send End Enable"=TRUE, "Message Based Settings:Termination Character"=w451) -> (reference out=w454:refnum<visa-resource-name>, error out=w453:errorcluster)
              }
            }
            n186 = while {
              shift-right: [w473] -> w428
              shift-left: w431 -> [w486]
              tunnel: w433 -> [w485]
              tunnel: [w472] -> w427
              stop <- w487 stop-if-true
              # "串口写入和读取循环"
              n187 = Number To Decimal String(number=-3000 ("数字")) -> (decimal integer string=w467:string)  [unwired: 1 in]
              n188 = Concatenate Strings("0x00 W 0x607A " ("字符串"), w467) -> (w483:string)
              n189 = VISA Write(VISA resource name=w486, write buffer=w483, error in (no error)=w485) -> (VISA resource name out=w470:refnum<visa-resource-name>, error out=w469:errorcluster)  [unwired: 1 out]
              n190 = property class="Instr"(reference=w470, error in=w469) -> (reference out=w478:refnum<visa-resource-name>, error out=w477:errorcluster, "Bytes at Port"=w476:u32)
              n191 = Wait (ms)(milliseconds to wait=u32 20 ("等待时间（毫秒）")) -> ()  [unwired: 1 out]
              n192 = VISA Read(VISA resource name=w478, byte count=w476, error in (no error)=w477) -> (VISA resource name out=w473:refnum<visa-resource-name>, read buffer=w475:string, error out=w472:errorcluster)  [unwired: 1 out]
              n193 = feedback #7("") -> (w481:string)
              n194 = Concatenate Strings(w481, w475) -> (w480:string)
              "坐标设定命令串口传输响应 3" <- w480
              n195 = feedback-in #7(w480) -> ()
              n196 = call <vilib>:"Trim Whitespace.vi"("string"=w475) -> ("trimmed string"=w474:string)  [unwired: 1 in]
              n197 = Concatenate Strings("0x00 W 0x607A ", w467) -> (w466:string)
              n198 = Equal?(x=w474, y=w466) -> (x = y?=w471:bool)
              n199 = Or(x=w472, y=w471) -> (x .or. y?=w487:bool)
            }
            n200 = VISA Close(VISA resource name=w428, error in (no error)=w427) -> ()  [unwired: 1 out]
          }
          frame #1 {
            n201 = flat-sequence {
              frame #0 {
                n202 = Unbundle By Name("XON/XOFF字符 6") -> ("XON"=w495:T2, "XOFF"=w494:T2)
                n203 = Unbundle By Name(T3 {"波特率"=115200, "数据比特"=8, "奇偶"=enum."None", "停止位"=10, "流控制"=0} ("串口设置")) -> ("波特率"=w499:u32, "数据比特"=w500:u16, "奇偶"=w501:enum16{"None", "Odd", "Even", "Mark", "Space"}, "停止位"=w502:u16, "流控制"=w496:u16)
                n204 = call-poly "VISA Configure Serial Port"("VISA resource name"=refnum<visa-resource-name> "COM3" ("VISA资源名称"), "termination char\n(0xA = '\\n' = LF)"="终止符 6", "Enable Termination\nChar (T)"="终止符时结束读取？ 6", "baud rate (9600)"=w499, "data bits (8)"=w500, "parity (0:none)"=w501, "stop bits (10: 1 bit)"=w502, "flow control (0:none)"=w496) -> ("VISA resource name out"=w503:refnum<visa-resource-name>, "error out"=w504:errorcluster)  [unwired: 2 in, 4 out]
                n205 = case shown="1" w496 {
                  tunnel: [w518 w525] -> w493
                  tunnel: [w519 w524] -> w492
                  tunnel: w504 -> [w518 w523]
                  tunnel: w503 -> [w519 w522]
                  tunnel: w495 -> [_ w521]
                  tunnel: w494 -> [_ w520]
                  frame Default {
                  }
                  frame 1 {
                    n206 = property class="Instr"(reference=w522, error in=w523, "Serial Settings:Flow Control XON Character"=w521, "Serial Settings:Flow Control XOFF Character"=w520) -> (reference out=w524:refnum<visa-resource-name>, error out=w525:errorcluster)
                  }
                }
                n207 = case shown="真" "终止符时结束写入？ 6" {
                  tunnel: w492 -> [w509 w517]
                  tunnel: w493 -> [w510 w516]
                  tunnel: [w509 w515] -> w489
                  tunnel: [w510 w514] -> w488
                  tunnel: "终止符 6" -> [_ w512]
                  frame False {
                  }
                  frame True {
                    w513 = u16 2 items=["None", "LastBit", "TermChar", "Break"] ("Serial Settings:Serial End Mode for Writes")
                    n208 = property class="Instr"(reference=w517, error in=w516, "Serial Settings:End Mode for Writes"=w513, "Message Based Settings:Send End Enable"=TRUE, "Message Based Settings:Termination Character"=w512) -> (reference out=w515:refnum<visa-resource-name>, error out=w514:errorcluster)
                  }
                }
                n209 = while {
                  shift-right: [w545] -> w508
                  shift-left: w489 -> [w544]
                  tunnel: w488 -> [w543]
                  tunnel: [w541] -> w507
                  stop <- w530 stop-if-true
                  # "串口写入和读取循环"
                  n210 = VISA Write(VISA resource name=w544, write buffer="0x00 W 0x12C04 5" ("写入缓冲区"), error in (no error)=w543) -> (VISA resource name out=w535:refnum<visa-resource-name>, error out=w532:errorcluster)  [unwired: 1 out]
                  n211 = property class="Instr"(reference=w535, error in=w532) -> (reference out=w534:refnum<visa-resource-name>, error out=w533:errorcluster, "Bytes at Port"=w531:u32)
                  n212 = Wait (ms)(milliseconds to wait=u32 10) -> ()  [unwired: 1 out]
                  n213 = VISA Read(VISA resource name=w534, byte count=w531, error in (no error)=w533) -> (VISA resource name out=w545:refnum<visa-resource-name>, read buffer=w528:string, error out=w541:errorcluster)  [unwired: 1 out]
                  n214 = feedback #8("") -> (w539:string)
                  n215 = Concatenate Strings(w539, w528) -> (w538:string)
                  "运动命令执行串口响应 3" <- w538
                  n216 = feedback-in #8(w538) -> ()
                  n217 = call <vilib>:"Trim Whitespace.vi"("string"=w528) -> ("trimmed string"=w527:string)  [unwired: 1 in]
                  n218 = Equal?(x=w527, y="0x00 W 0x12C04 5") -> (x = y?=w526:bool)
                  n219 = Or(x=w526, y="停止 5") -> (x .or. y?=w530:bool)
                }
                n220 = VISA Close(VISA resource name=w508, error in (no error)=w507) -> ()  [unwired: 1 out]
              }
            }
          }
        }
      }
    }
  }
